vi "FTW-CodeGen-GetTerms.vi"(0 "State In":T3 {"Actor Interface"."Bounds"."Left" format="%dpx"; "Actor Interface"."Bounds"."Top" format="%dpx"; "Actor Interface"."Bounds"."Right" format="%dpx"; "Actor Interface"."Bounds"."Bottom" format="%dpx"}, 5 "XRef":refnum<vi>) -> (4 "Terms":T2(array[cluster]), 6 "Actor Terminals":T1(array[cluster]))   [LabVIEW 2015, in "FTW-Actor-Spawn.xnode"]
uses:
  FTW-Actor-Spawn.xnode
  FTW-CodeGen-State.ctl
panel:
  # "Inputs"
  # "Outputs"
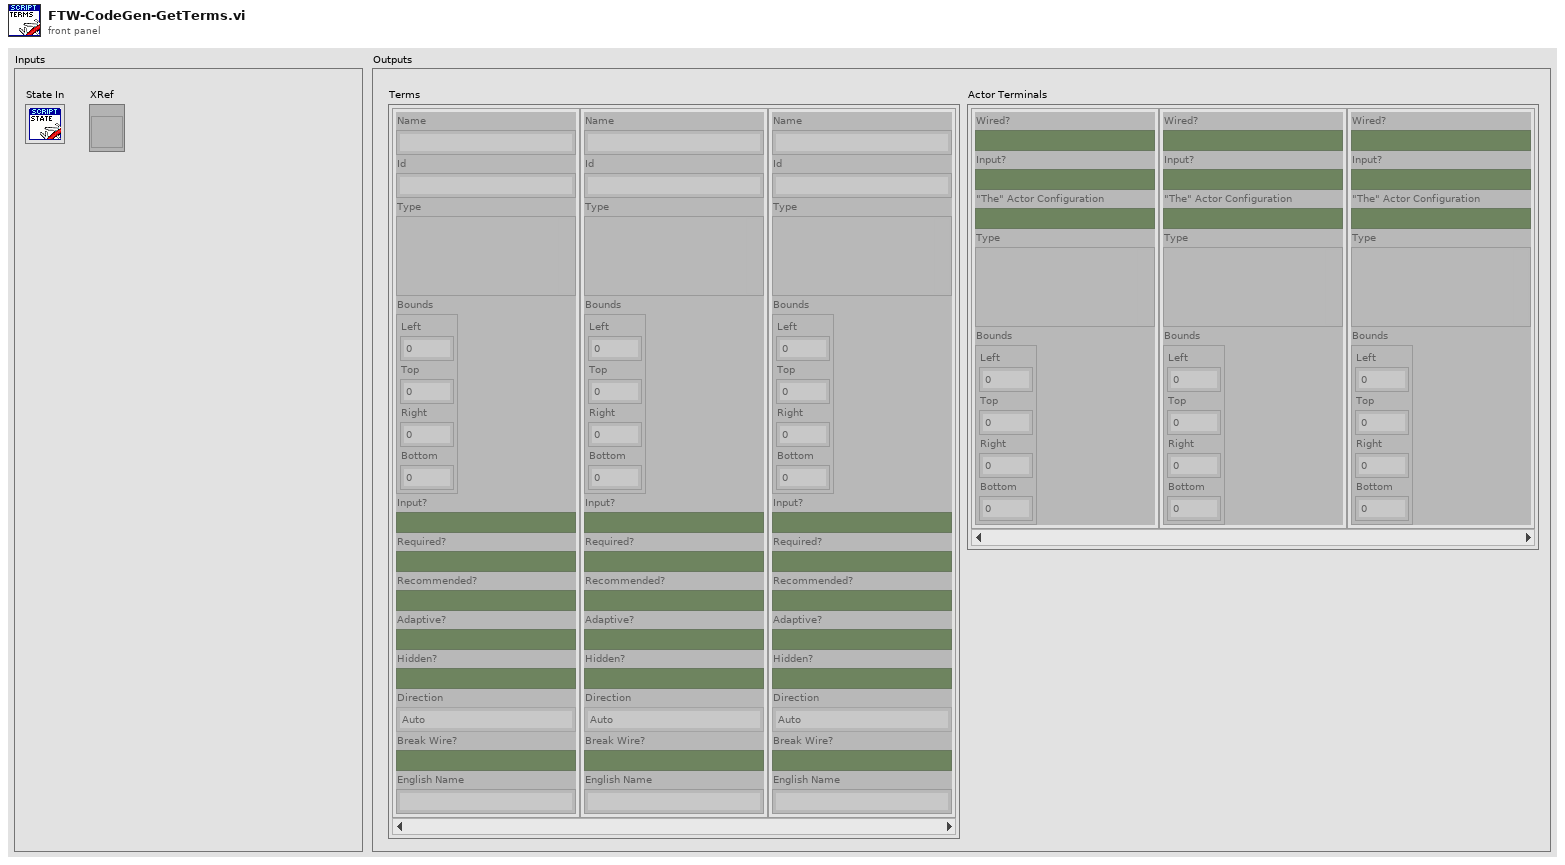
[diagram p1: front panel]
types:
  T1 = cluster{"Wired?":bool, "Input?":bool, "\"The\" Actor Configuration":bool, "Type":variant, "Bounds":cluster{"Left":i32, "Top":i32, "Right":i32, "Bottom":i32}}[]
  T2 = cluster{"Name":string, "Id":string, "Type":variant, "Bounds":cluster{"Left":i32, "Top":i32, "Right":i32, "Bottom":i32}, "Input?":bool, "Required?":bool, "Recommended?":bool, "Adaptive?":bool, "Hidden?":bool, "Direction":enum32{"Auto", "Up", "Down", "Left", "Right", "Center"}, "Break Wire?":bool, "English Name":string}[]
  T3 = typedef "FTW-Actor-Spawn.xnode/FTW-CodeGen-State.ctl" = cluster{"Path Wired?":bool, "Actor Interface":cluster{"Name":string, "Type":variant, "Bounds":cluster{"Left":i32, "Top":i32, "Right":i32, "Bottom":i32}, "Input":bool, "Recommended":bool, "Required":bool, "Dynamic Dispatch":bool, "On Interface":bool, "\"The\" Config Terminal":bool}[], "Config Terminal Index":i32}
  T4 = cluster{"Name":string, "Type":variant, "Bounds":cluster{"Left":i32, "Top":i32, "Right":i32, "Bottom":i32}, "Input":bool, "Recommended":bool, "Required":bool, "Dynamic Dispatch":bool, "On Interface":bool, "\"The\" Config Terminal":bool}[]
  T5 = cluster{"Name":string, "Id":string, "Type":variant, "Bounds":cluster{"Left":i32, "Top":i32, "Right":i32, "Bottom":i32}, "Input?":bool, "Required?":bool, "Recommended?":bool, "Adaptive?":bool, "Hidden?":bool, "Direction":enum32{"Auto", "Up", "Down", "Left", "Right", "Center"}, "Break Wire?":bool, "English Name":string}
  T6 = cluster{"Wired?":bool, "Input?":bool, "\"The\" Actor Configuration":bool, "Type":variant, "Bounds":cluster{"Left":i32, "Top":i32, "Right":i32, "Bottom":i32}}
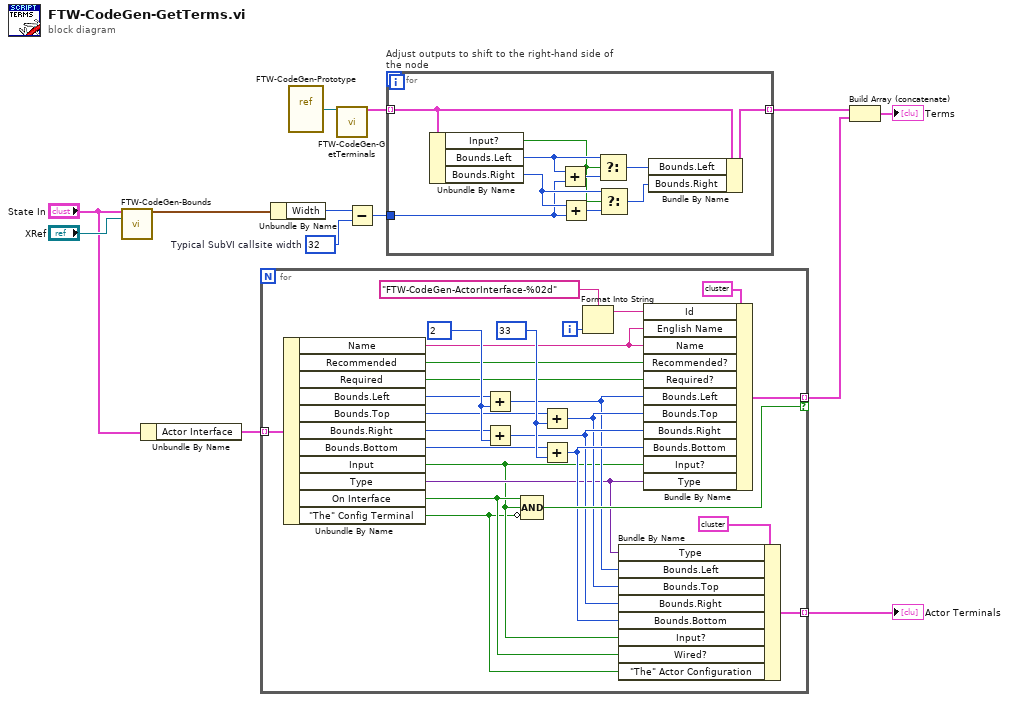
[diagram p0: block diagram]
diagram:
  w6 = 32  # Typical SubVI callsite width
  n1 = call "FTW-CodeGen-Bounds.vi"("State In"="State In", "XRef"="XRef") -> ("Bounds"=w8:cluster{"Width":i32, "Height":i32})  [unwired: 13 in]
  n2 = Unbundle By Name("State In") -> ("Actor Interface"=w2:T4)
  n3 = for {
    tunnel: [w39] -> w12 mode=indexing if=w30
    tunnel: [w33] -> w11 mode=indexing
    tunnel: w2 -> [w19] mode=indexing
    i -> [w18]
    w37 = 33 ("y")
    w38 = 2 ("y")
    n4 = Unbundle By Name(w19) -> ("Name"=w36:string, "Recommended"=w35:bool, "Required"=w34:bool, "Bounds.Left"=w28:i32, "Bounds.Top"=w27:i32, "Bounds.Right"=w26:i32, "Bounds.Bottom"=w25:i32, "Input"=w15:bool, "Type"=w20:variant, "On Interface"=w31:bool, "\"The\" Config Terminal"=w14:bool)
    n5 = Add(x=w28, y=w38) -> (x+y=w21:i32)
    n6 = Add(x=w26, y=w38) -> (x+y=w23:i32)
    n7 = Compound Arithmetic op=AND(w31, w15, invert w14) -> (w30:bool)
    n8 = Add(x=w27, y=w37) -> (x+y=w22:i32)
    n9 = Add(x=w25, y=w37) -> (x+y=w24:i32)
    n10 = Format Into String(format string="FTW-CodeGen-ActorInterface-%02d", w18) -> (resulting string=w17:string)  [unwired: 2 in, 1 out]
    n11 = Bundle By Name(cluster=T6 {"Wired?"=FALSE, "Input?"=FALSE, "\"The\" Actor Configuration"=FALSE, "Type"=variant, "Bounds"={"Left"=0, "Top"=0, "Right"=0, "Bottom"=0}} ("Term 4"), "Type"=w20, "Bounds.Left"=w21, "Bounds.Top"=w22, "Bounds.Right"=w23, "Bounds.Bottom"=w24, "Input?"=w15, "Wired?"=w31, "\"The\" Actor Configuration"=w14) -> (w33:T6)
    n12 = Bundle By Name(cluster=T5 {"Name"="", "Id"="", "Type"=variant, "Bounds"={"Left"=0, "Top"=0, "Right"=0, "Bottom"=0}, "Input?"=FALSE, "Required?"=FALSE, "Recommended?"=FALSE, "Adaptive?"=FALSE, "Hidden?"=FALSE, "Direction"=enum."Auto", "Break Wire?"=FALSE, "English Name"=""} ("Term 4"), "Id"=w17, "English Name"=w36, "Name"=w36, "Recommended?"=w35, "Required?"=w34, "Bounds.Left"=w21, "Bounds.Top"=w22, "Bounds.Right"=w23, "Bounds.Bottom"=w24, "Input?"=w15, "Type"=w20) -> (w39:T5)
  }
  "Actor Terminals" <- w11
  n13 = Unbundle By Name(w8) -> ("Width"=w7:i32)
  n14 = vi-ref "FTW-CodeGen-Prototype.vi"() -> (w1:refnum<vi>)
  n15 = call "FTW-CodeGen-GetTerminals.vi"("PrototypeVI"=w1) -> ("Terms"=w10:T2)  [unwired: 13 in, 1 out]
  n16 = Subtract(x=w7, y=w6) -> (x-y=w5:i32)
  n17 = for "Adjust outputs to shift to the right-hand side of the node" {
    tunnel: w10 -> [w49] mode=indexing
    tunnel: [w48] -> w9 mode=indexing
    tunnel: w5 -> [w40]
    n18 = Unbundle By Name(w49) -> ("Input?"=w41:bool, "Bounds.Left"=w46:i32, "Bounds.Right"=w43:i32)
    n19 = Add(x=w46, y=w40) -> (x+y=w45:i32)
    n20 = Add(x=w43, y=w40) -> (x+y=w44:i32)
    n21 = Select(t=w46, s=w41, f=w45) -> (s? t:f=w47:i32)
    n22 = Select(t=w43, s=w41, f=w44) -> (s? t:f=w42:i32)
    n23 = Bundle By Name(cluster=w49, "Bounds.Left"=w47, "Bounds.Right"=w42) -> (w48:T5)
  }
  n24 = Build Array (concatenate)(w9, w12) -> (→"Terms":T2)
